vi "Initialize.vi"(5 "TimingEngine":T1, 6 "Cfg wChassis":T2, 7 "LS DAQ Task":refnum<class "DAQ Task.lvclass">, 8 "error in (no error)":errorcluster, 9 "TCP LS Writer":refnum<class "Message Enqueuer.lvclass">, 10 "TCP HS Writer":refnum<class "Message Enqueuer.lvclass">, 11 "DAQ Actor in":refnum<class "DAQ Actor.lvclass">) -> (0 "error out":errorcluster, 3 "DAQ Actor out":refnum<class "DAQ Actor.lvclass">)   [LabVIEW 2018, in "Data Acquisition.lvlib" / "DAQ Actor.lvclass"]
uses:
  DAQ Actor.lvclass
  Class DAQ Task/DAQ Task.lvclass
  Custom Ctrls/Master Cfg/ge_Cfg wChassis.ctl
  Cfg Grandmaster/Class Chassis BOM/Chassis BOM.lvclass
  Cfg Grandmaster/Class Chassis Cfg/ChassisCfg.lvclass
  Class Chassis Tasks/Chassis Tasks.lvclass
  Common/Controls/TE_Designator.ctl
  <vilib>/ActorFramework/Message Enqueuer/Message Enqueuer.lvclass
  Cfg Grandmaster/Class Chassis BOM/Chassis BOM.lvclass/Chassis BOM.ctl
  DAQ Actor.lvclass/DAQ Actor.ctl
  Cfg Grandmaster/Class Chassis BOM/Read Chassis Alias.vi
  Cfg Grandmaster/Class Chassis BOM/Read IP Address.vi
  Cfg Grandmaster/Class Timing Group/Read Modbus URL.vi
  Cfg Grandmaster/Class Timing Group/TimingGrp.lvclass
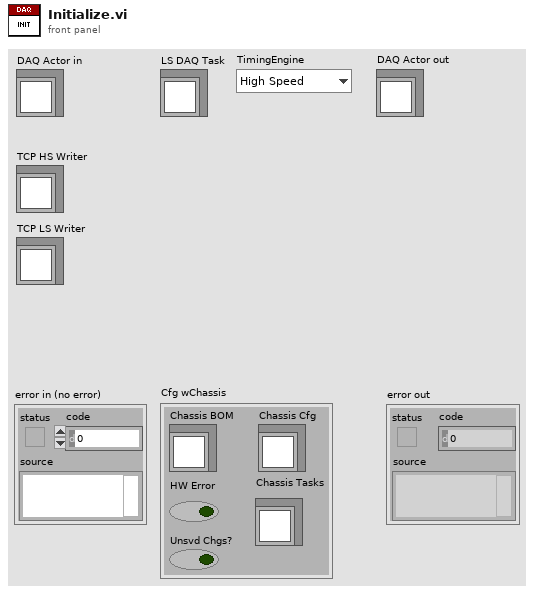
[diagram p1: front panel]
types:
  T1 = typedef "TE_Designator.ctl" = enum16{"High Speed", "Low Speed"}
  T2 = typedef "ge_Cfg wChassis.ctl" = cluster{"Chassis BOM":refnum<class "Chassis BOM.lvclass">, "Chassis Cfg":refnum<class "ChassisCfg.lvclass">, "Chassis Tasks":refnum<class "Chassis Tasks.lvclass">, "HW Error":bool, "Unsvd Chgs?":bool}
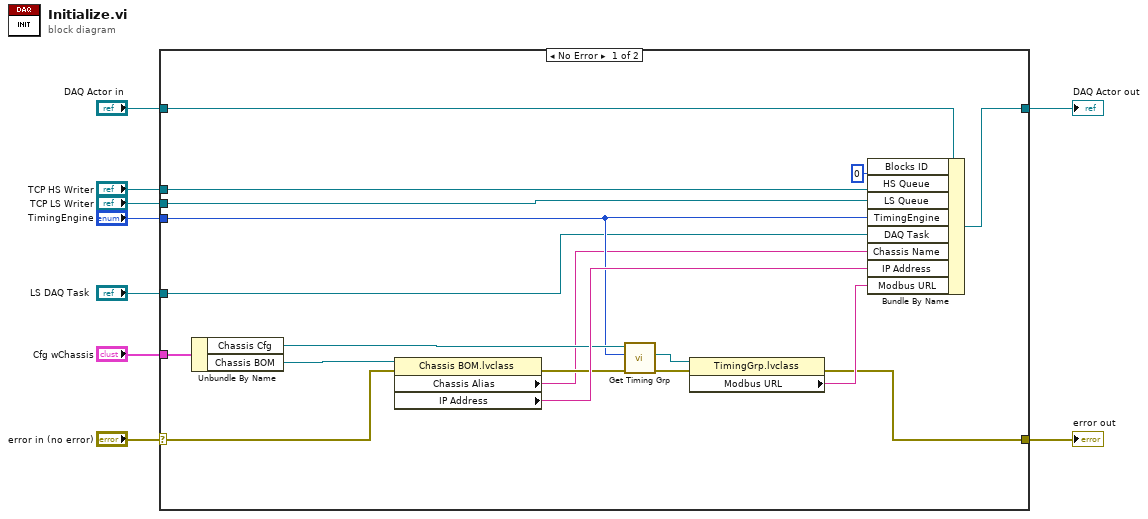
[diagram p0: block diagram]
diagram:
  n1 = case shown="No Error" "error in (no error)" {
    selector: "error in (no error)" -> [w12 w29]
    tunnel: [w14 w29] -> w8
    tunnel: [w15 w28] -> w6
    tunnel: "DAQ Actor in" -> [w17 w28]
    tunnel: "LS DAQ Task" -> [w13 _]
    tunnel: "TimingEngine" -> [w21 _]
    tunnel: "Cfg wChassis" -> [w26 _]
    tunnel: "TCP LS Writer" -> [w11 _]
    tunnel: "TCP HS Writer" -> [w10 _]
    frame No Error {
      n2 = Unbundle By Name(w26) -> ("Chassis Cfg"=w22:refnum<class "ChassisCfg.lvclass">, "Chassis BOM"=w25:refnum<class "Chassis BOM.lvclass">)
      n3 = property class="Chassis BOM.lvclass"(reference=w25, error in=w12) -> (error out=w23:errorcluster, "Chassis Alias"=w16:string, "IP Address"=w24:string)  [unwired: 1 out]
      n4 = call "Get Timing Grp.vi"("error in (no error)"=w23, "Timing Engine"=w21, "Chassis Cfg"=w22) -> ("error out"=w19:errorcluster, "Timing Groups"=w20:refnum<class "TimingGrp.lvclass">)  [unwired: 6 in, 1 out]
      n5 = property class="TimingGrp.lvclass"(reference=w20, error in=w19) -> (error out=w14:errorcluster, "Modbus URL"=w18:string)  [unwired: 1 out]
      n6 = Bundle By Name(cluster=w17, "Blocks ID"=u32 0, "HS Queue"=w10, "LS Queue"=w11, "TimingEngine"=w21, "DAQ Task"=w13, "Chassis Name"=w16, "IP Address"=w24, "Modbus URL"=w18) -> (w15:refnum<class "DAQ Actor.lvclass">)
    }
    frame Error {
    }
  }
  "error out" <- w8
  "DAQ Actor out" <- w6
